vi "LC Language Demo.vi"() -> ()   [LabVIEW 2020]
uses:
  SubVI/LC Language.ctl
  SubVI/LC Single Control Information.ctl
  SubVI/LC Mode.ctl
  SubVI/LC Global Mode.ctl
panel:
  in  "Title":string="Language Change System"
  in  "Path":path
  in  "VI Path":string(tree)
  in  "Control Path":string(tree)
  in  "Import":bool
  in  "Export":bool
  in  "Class ID":u32
  in  "Control Type":string
  in  "Add":bool
  in  "Language":T1 items=["Chinese", "English"]
  in  "Property":u16(ring) items=["Blinking", "BoolText.Text", "Caption.Position", "Caption.Text", "Caption.Visible", "DefVal", "Desc", "FP.Title", "Lable.Text", "Lable.Visible", "Strings[4]", "TipStrip", "VI_Desc", "Visible"]
  in  "Control Ref":string
  in  "Control_Info":T2
  in  "Control List":i32(listbox)
  out "Time":string
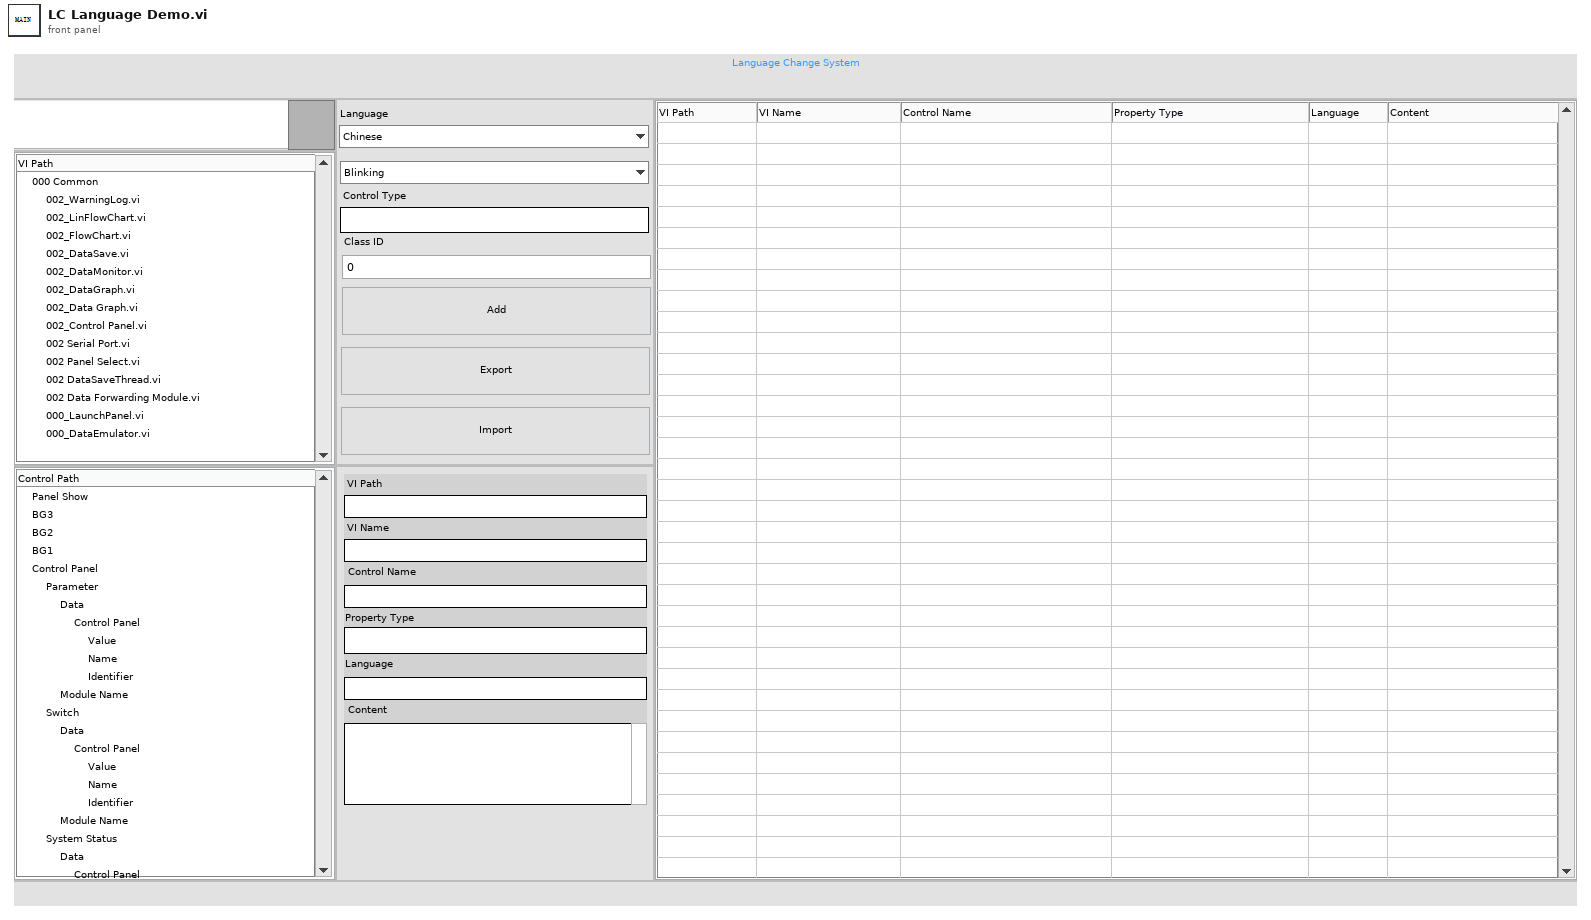
[diagram p1: front panel]
types:
  T1 = typedef "LC Language.ctl" = u16
  T2 = typedef "LC Single Control Information.ctl" = cluster{"VI Path":string, "VI Name":string, "Control Name":string, "Property Type":string, "Language":string, "Content":string}
  T3 = typedef "LC Global Mode.ctl" = enum16{"Init", "Read", "Write Language", "Write Version", "Save"}
  T4 = typedef "LC Mode.ctl" = enum16{"Init", "NONE", "Read", "Write", "Delete", "Clear", "Save"}
  T5 = typedef "LVPoint32TypeDef.ctl" = cluster{"Horizontal":i32, "Vertical":i32}
  T6 = typedef "LVRowAndColumnTypeDef.ctl" = cluster{"Row":i32, "Column":i32}
  T7 = enum32{"invalid app kind", "Development System", "Run Time System", "Student Edition", "Embedded LabVIEW", "Evaluation", "Custom"}
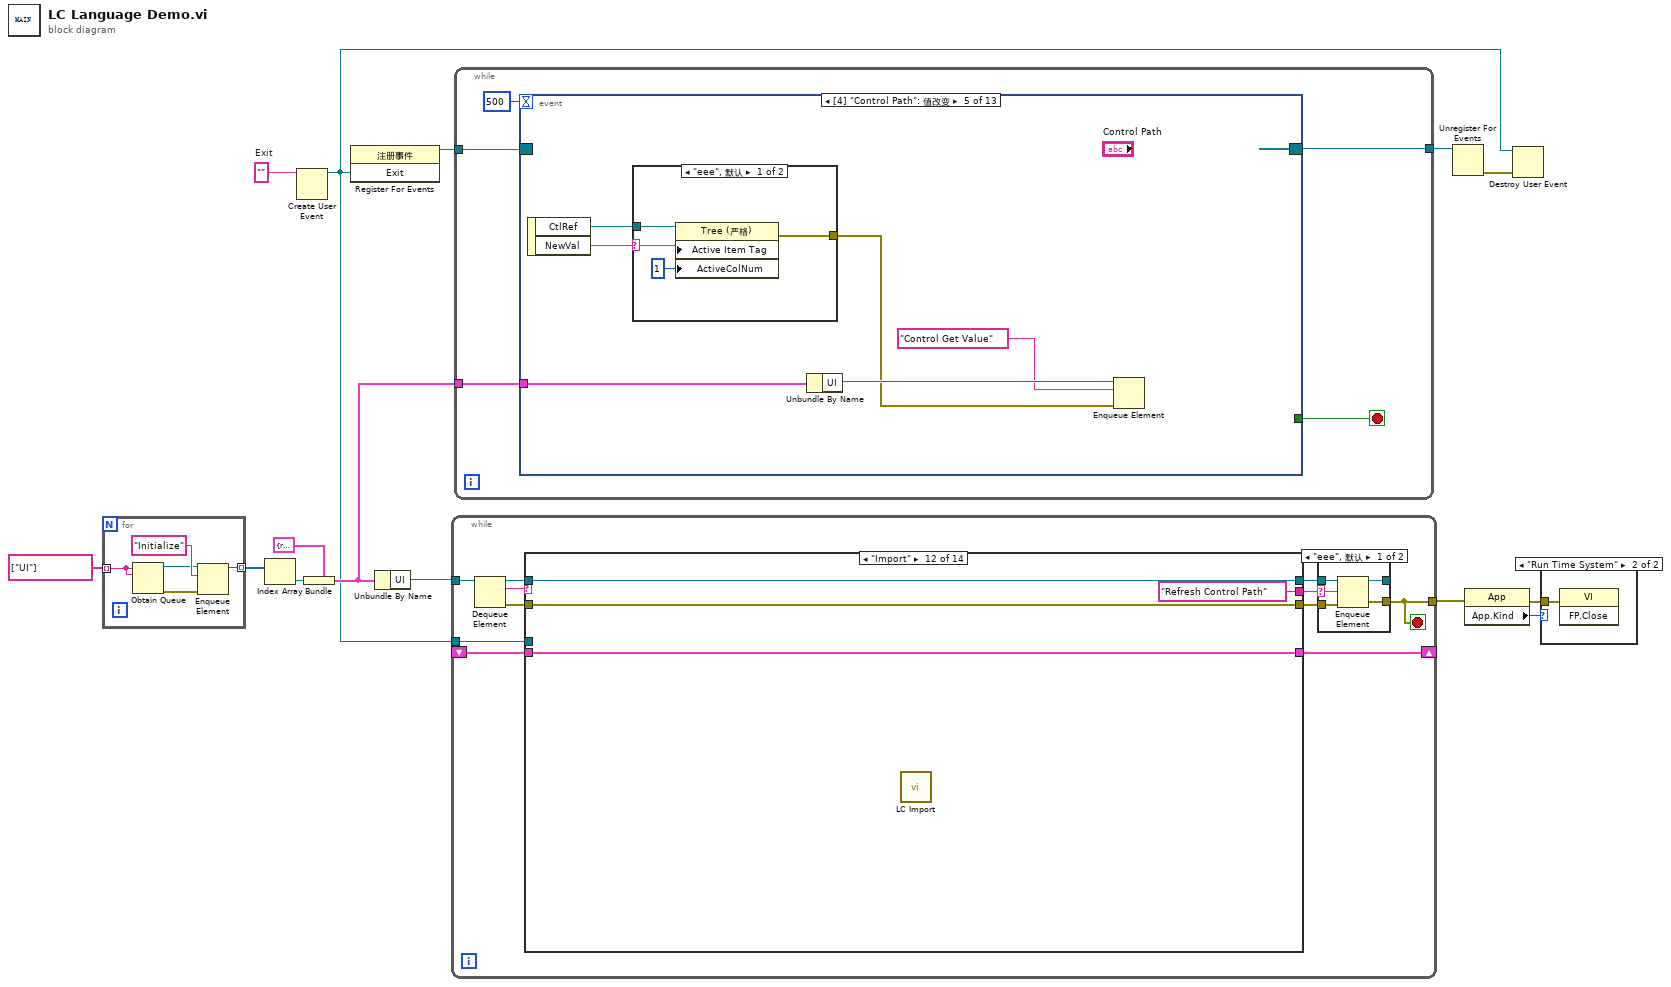
[diagram p0: block diagram]
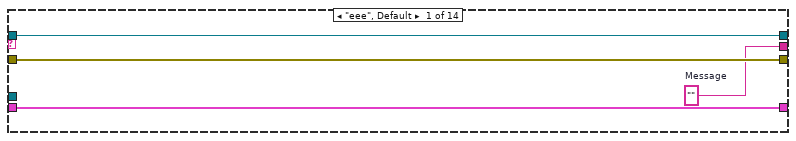
[diagram p4: hidden frame]
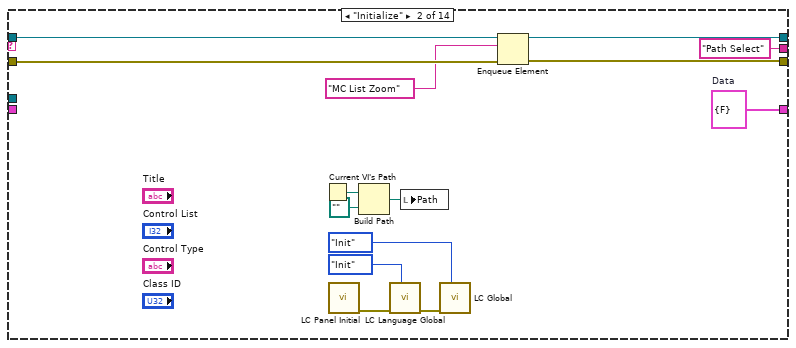
[diagram p5: hidden frame]
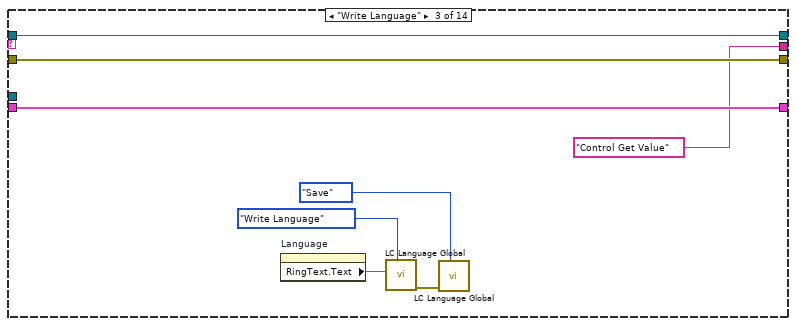
[diagram p6: hidden frame]
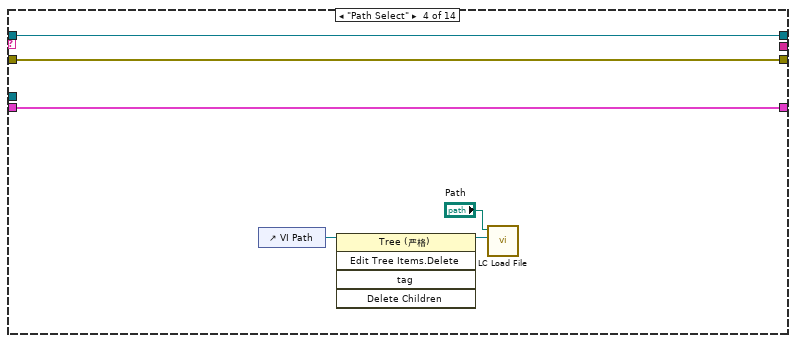
[diagram p7: hidden frame]
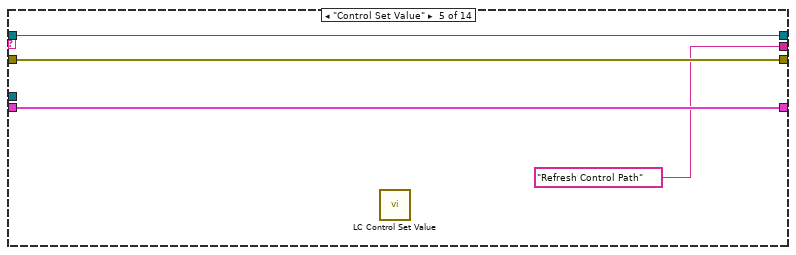
[diagram p8: hidden frame]
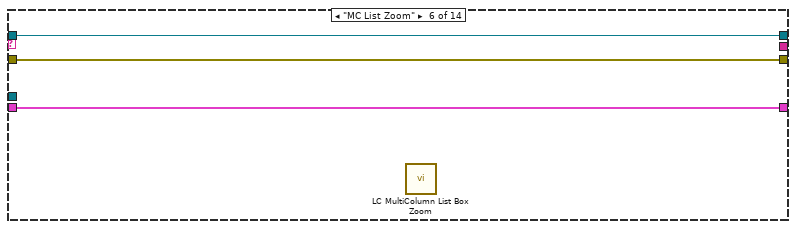
[diagram p9: hidden frame]
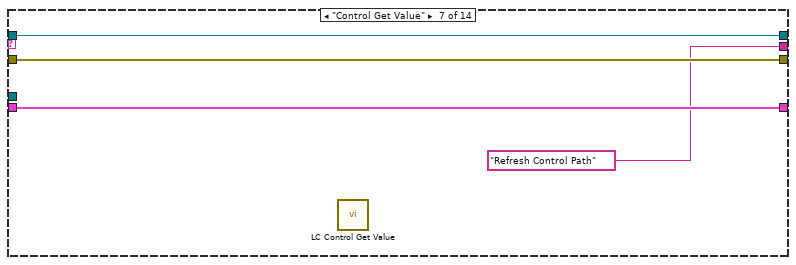
[diagram p10: hidden frame]
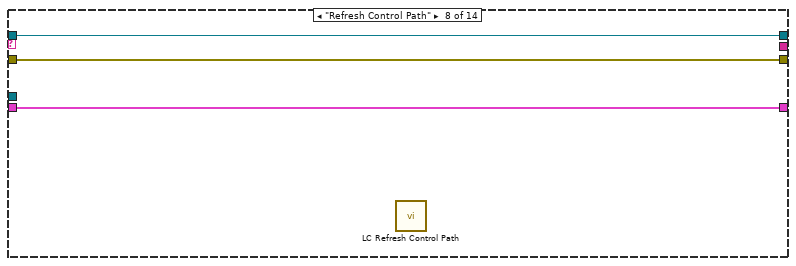
[diagram p11: hidden frame]
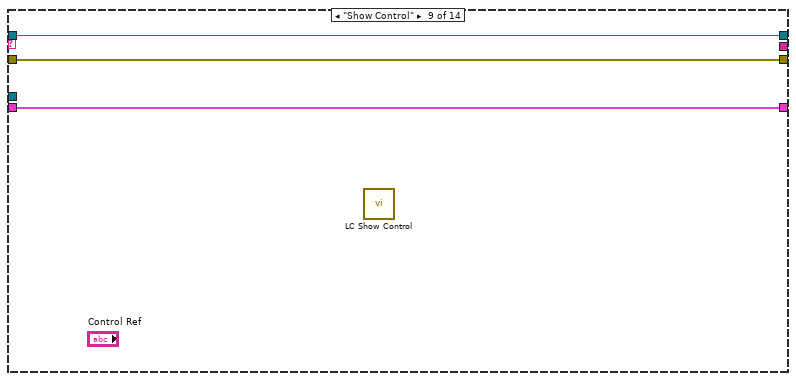
[diagram p12: hidden frame]
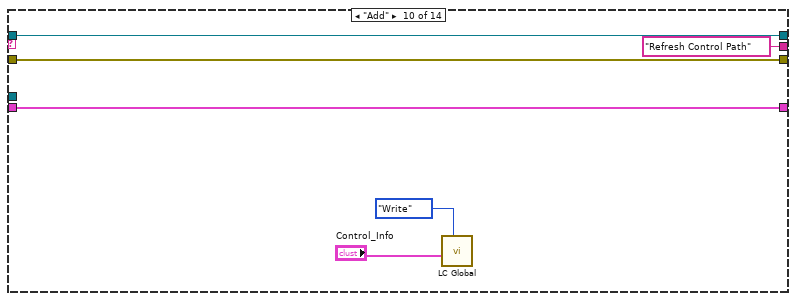
[diagram p13: hidden frame]
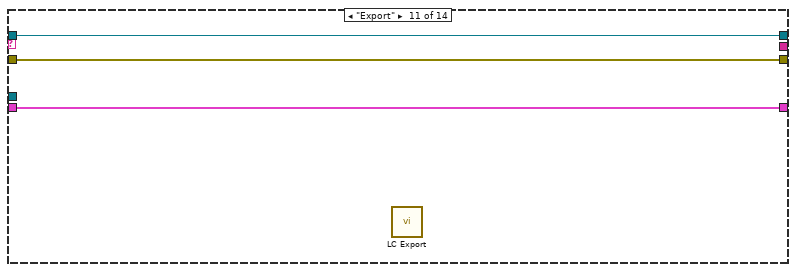
[diagram p14: hidden frame]
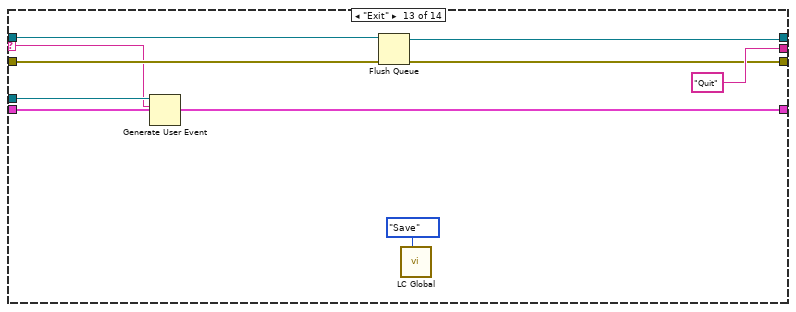
[diagram p15: hidden frame]
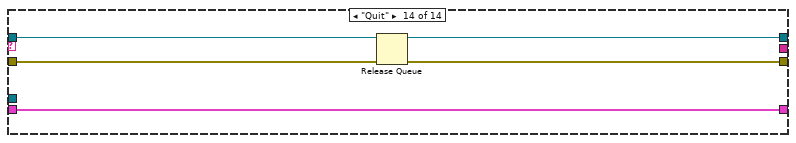
[diagram p16: hidden frame]
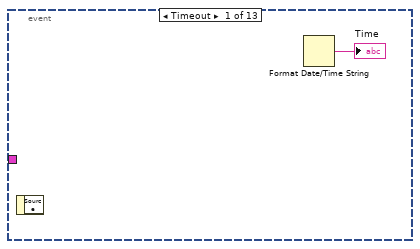
[diagram p17: hidden frame]
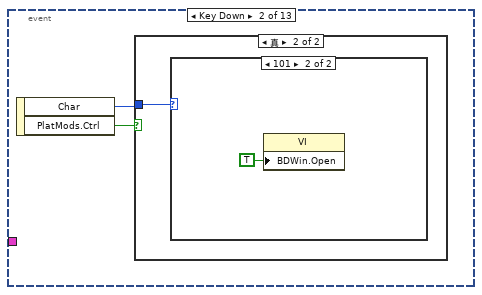
[diagram p18: hidden frame]
diagram:
  w4 = ""  # Exit
  n1 = for {
    tunnel: string[] ["UI"] -> [w15] mode=indexing
    tunnel: [w16] -> w9 mode=indexing
    n2 = Obtain Queue(name (unnamed)=w15, element data type=w15) -> (queue out=w18:refnum<queue>, error out=w17:errorcluster)  [unwired: 3 in, 1 out]
    n3 = Enqueue Element(queue=w18, element="Initialize" ("元素"), error in (no error)=w17) -> (queue out=w16:refnum<queue>)  [unwired: 1 in, 2 out]
  }
  n4 = Index Array(array=w9) -> (element=w13:refnum<queue>)  [unwired: 1 in]
  n5 = Create User Event(user event datatype=w4) -> (user event=w8:refnum<user-event>)  [unwired: 1 in, 1 out]
  n6 = Bundle(cluster=cluster{"UI":refnum<queue>} {"UI"=refnum}, "UI"=w13) -> (w14:cluster{"UI":refnum<queue>})
  n7 = register-events(w8) -> (reference out=w5:refnum<event-registration>)  [unwired: 2 in, 1 out]
  n8 = Unbundle By Name(w14) -> ("UI"=w10:refnum<queue>)
  n9 = while {
    tunnel: w10 -> [w30]
    tunnel: [w20] -> w1
    shift-right: [w24] -> _
    shift-left: _ -> [w23]
    tunnel: w8 -> [w22]
    stop <- w20 stop-if-true
    n10 = Dequeue Element(queue=w30) -> (queue out=w29:refnum<queue>, element=w21:string, error out=w26:errorcluster)  [unwired: 2 in, 1 out]
    n11 = case shown="\"Import\"" w21 {
      selector: w21 -> [_ _ _ _ _ _ _ _ _ _ _ _ w101 _]
      tunnel: w29 -> [w41 w47 w63 w69 w73 w76 w80 w83 w86 w92 w95 w99 w106 w112]
      tunnel: [w41 w44 w63 w69 w73 w76 w80 w83 w86 w92 w95 w99 w105 w112] -> w28
      tunnel: [w40 w43 w62 w68 w72 w75 w79 w82 w85 w91 w94 w98 w104 w109] -> w27
      tunnel: w26 -> [w40 w46 w62 w68 w72 w75 w79 w82 w85 w91 w94 w98 w103 w111]
      tunnel: [w39 "Path Select" ("Message") "Control Get Value" ("Message") _ "Refresh Control Path" ("Message") _ "Refresh Control Path" ("Message") _ _ "Refresh Control Path" ("Message") _ "Refresh Control Path" ("Message") "Quit" ("Message") _] -> w25
      tunnel: [w38 w55 w61 w67 w71 w74 w78 w81 w84 w90 w93 w97 w108 w110] -> w24
      tunnel: w23 -> [w38 _ w61 w67 w71 w74 w78 w81 w84 w90 w93 w97 w108 w110]
      tunnel: w22 -> [_ _ _ _ _ _ _ _ _ _ _ _ w102 _]
      frame "eee", Default {
        w39 = ""  # Message
      }
      frame "Initialize" {
        w55 = cluster{"Data":bool} {"Data"=FALSE}  # Data
        n12 = Current VI's Path() -> (path=w53:path)
        n13 = call "LC Panel Initial.vi"() -> ("error out"=w50:errorcluster)  [unwired: 11 in]
        n14 = Build Path(base path=w53, name or relative path=path ".." ("名称或相对路径")) -> (appended path=w51:path)
        n15 = call "LC Language Global.vi"("Mode"=LC_Global_Mode."Init", "error in (no error)"=w50) -> ("error out"=w49:errorcluster)  [unwired: 8 in, 1 out]
        n16 = local write "Path"(w51) -> ()
        n17 = call "LC Global.vi"("Mode"=LC_Mode."Init", "error in (no error)"=w49) -> ()  [unwired: 7 in, 3 out]
        n18 = Enqueue Element(queue=w47, element="MC List Zoom" ("元素"), error in (no error)=w46) -> (queue out=w44:refnum<queue>, error out=w43:errorcluster)  [unwired: 1 in, 1 out]
      }
      frame "Write Language" {
        n19 = property on="Language" class="Ring (严格)"() -> ("RingText.Text"=w59:string)  [unwired: 2 in, 2 out]
        n20 = call "LC Language Global.vi"("Mode"=LC_Global_Mode."Write Language", "String In"=w59) -> ("error out"=w57:errorcluster)  [unwired: 8 in, 1 out]
        n21 = call "LC Language Global.vi"("Mode"=LC_Global_Mode."Save", "error in (no error)"=w57) -> ()  [unwired: 8 in, 2 out]
      }
      frame "Path Select" {
        n22 = control-ref of="VI Path"() -> (w66:refnum<vi>)
        n23 = invoke class="Tree (严格)" method="Edit Tree Items.Delete"(reference=w66) -> (reference out=w65:refnum<vi>)  [unwired: 4 in, 4 out]
        n24 = call "LC Load File.vi"("VI Path"=w65, "selected path"="Path") -> ()  [unwired: 9 in, 1 out]
      }
      frame "Control Set Value" {
        n25 = call "LC Control Set Value.vi"() -> ()  [unwired: 11 in, 1 out]
      }
      frame "MC List Zoom" {
        n26 = call "LC MultiColumn List Box Zoom.vi"() -> ()  [unwired: 11 in, 1 out]
      }
      frame "Control Get Value" {
        n27 = call "LC Control Get Value.vi"() -> ()  [unwired: 11 in, 1 out]
      }
      frame "Refresh Control Path" {
        n28 = call "LC Refresh Control Path.vi"() -> ()  [unwired: 11 in, 1 out]
      }
      frame "Show Control" {
        n29 = call "LC Show Control.vi"() -> ()  [unwired: 11 in, 1 out]
      }
      frame "Add" {
        n30 = call "LC Global.vi"("Mode"=LC_Mode."Write", "Write"="Control_Info") -> ()  [unwired: 7 in, 3 out]
      }
      frame "Export" {
        n31 = call "LC Export.vi"() -> ()  [unwired: 11 in, 1 out]
      }
      frame "Import" {
        n32 = call "LC Import.vi"() -> ()  [unwired: 11 in, 1 out]
      }
      frame "Exit" {
        n33 = Generate User Event(user event=w102, event data cluster=w101) -> ()  [unwired: 2 in, 2 out]
        n34 = Flush Queue(queue=w106, error in (no error)=w103) -> (queue out=w105:refnum<queue>, error out=w104:errorcluster)  [unwired: 1 out]
        n35 = call "LC Global.vi"("Mode"=LC_Mode."Save") -> ()  [unwired: 8 in, 3 out]
      }
      frame "Quit" {
        n36 = Release Queue(queue=w112, error in (no error)=w111) -> (error out=w109:errorcluster)  [unwired: 1 in, 2 out]
      }
    }
    n37 = case shown="\"eee\", 默认" w25 {
      selector: w25 -> [w31 _]
      tunnel: w28 -> [w35 w37]
      tunnel: w27 -> [w34 w36]
      tunnel: [w33 w36] -> w20
      tunnel: [w32 w37] -> _
      frame "eee", Default {
        n38 = Enqueue Element(queue=w35, element=w31, error in (no error)=w34) -> (queue out=w32:refnum<queue>, error out=w33:errorcluster)  [unwired: 1 in, 1 out]
      }
      frame "" {
      }
    }
  }
  n39 = while {
    tunnel: w5 -> [w116]
    tunnel: [w115] -> w7
    tunnel: w14 -> [w114]
    stop <- w117 stop-if-true
    n40 = event shown="[4] \"Control Path\": 值改变" {
      selector: w116 -> [_ _ _ _ _ _ _ _ _ _ _ _ _]
      dyn-events: [_ _ _ _ _ _ _ _ _ _ _ _ _] -> w115
      timeout: 500 -> [_ _ _ _ _ _ _ _ _ _ _ _ _]
      tunnel: [_ _ w124 w129 _ _ _ _ _ _ _ _ _] -> w117
      tunnel: w114 -> [_ _ _ w128 w133 w144 w147 w150 w151 w163 w166 w169 _]
      event Timeout {
        n41 = event-data() -> ()  [unwired: 1 in, 1 out]
        n42 = Format Date/Time String() -> (date/time string=→"Time":string)  [unwired: 3 in]
      }
      event Key Down {
        n43 = event-data() -> ("Char"=w120:i16, "PlatMods.Ctrl"=w119:bool)  [unwired: 1 in]
        n44 = case shown="真" w119 {
          tunnel: w120 -> [_ w121]
          frame False {
          }
          frame True {
            n45 = case shown="101" w121 {
              frame 0, Default {
              }
              frame 101 {
                n46 = property class="VI"("BDWin.Open"=TRUE ("程序框图窗口:打开")) -> ()  [unwired: 2 in, 2 out]
              }
            }
          }
        }
      }
      event User Event {
        n47 = event-data() -> ("Exit"=w125:string)  [unwired: 1 in]
        n48 = Equal?(x=w125, y="Exit") -> (x = y?=w124:bool)
      }
      event Panel Close? {
        w129 = TRUE ("放弃？")
        n49 = event-data() -> ()  [unwired: 1 in, 1 out]
        n50 = Cluster To Array(cluster=w128) -> (array=w127:refnum<queue>[])
        n51 = for {
          tunnel: w127 -> [w131] mode=indexing
          tunnel: "Exit" ("元素") -> [w130]
          n52 = Enqueue Element(queue=w131, element=w130) -> ()  [unwired: 2 in, 3 out]
        }
        n53 = event-data("Discard?"=w129) -> ()  [unwired: 1 in, 1 out]
      }
      event "Control Path": Value Change {
        n54 = event-data() -> ("CtlRef"=w136:refnum<vi>, "NewVal"=w137:string)  [unwired: 1 in]
        n55 = case shown="\"eee\", 默认" w137 {
          selector: w137 -> [w139 _]
          tunnel: w136 -> [w140 _]
          tunnel: [w138 _] -> w132
          frame "eee", Default {
            n56 = property class="Tree (严格)"(reference=w140, "Active Item Tag"=w139, "ActiveColNum"=1 ("活动单元格:活动列数")) -> (error out=w138:errorcluster)  [unwired: 1 in, 1 out]
          }
          frame "" {
          }
        }
        n57 = Unbundle By Name(w133) -> ("UI"=w135:refnum<queue>)
        n58 = Enqueue Element(queue=w135, element="Control Get Value" ("元素"), error in (no error)=w132) -> ()  [unwired: 1 in, 3 out]
      }
      event "Path": Value Change {
        n59 = event-data() -> ()  [unwired: 1 in, 1 out]
        n60 = Unbundle By Name(w144) -> ("UI"=w143:refnum<queue>)
        n61 = Enqueue Element(queue=w143, element="Path Select" ("元素")) -> ()  [unwired: 2 in, 3 out]
      }
      event Value Change {
        n62 = event-data() -> ()  [unwired: 1 in, 6 out]
        n63 = Unbundle By Name(w147) -> ("UI"=w146:refnum<queue>)
        n64 = Enqueue Element(queue=w146, element="Control Set Value" ("元素")) -> ()  [unwired: 2 in, 3 out]
      }
      event Panel Resize {
        n65 = event-data() -> ()  [unwired: 1 in, 1 out]
        n66 = Unbundle By Name(w150) -> ("UI"=w149:refnum<queue>)
        n67 = Enqueue Element(queue=w149, element="MC List Zoom" ("元素")) -> ()  [unwired: 2 in, 3 out]
      }
      event "VI Path": Value Change {
        n68 = event-data() -> ("NewVal"=w156:string)  [unwired: 1 in]
        n69 = call <vilib>:"Delimited String to 1D String Array.vi"("delimiter"=".", "delimited string"=w156) -> ("string array"=w154:string[])  [unwired: 9 in]
        n70 = Index Array(array=w154, index=1 ("索引")) -> (element=w152:string)
        n71 = case shown="\"vi\"" w152 {
          tunnel: w151 -> [_ w159]
          frame "eee", Default {
          }
          frame "vi" {
            n72 = Unbundle By Name(w159) -> ("UI"=w158:refnum<queue>)
            n73 = Enqueue Element(queue=w158, element="Refresh Control Path" ("元素")) -> ()  [unwired: 2 in, 3 out]
          }
        }
      }
      event "Add", "Export", "Import": Value Change {
        n74 = event-data() -> ("CtlRef"=w161:refnum<vi>)  [unwired: 1 in]
        n75 = Unbundle By Name(w163) -> ("UI"=w162:refnum<queue>)
        n76 = property class="Bool"(reference=w161) -> ("Label.Text"=w160:string)  [unwired: 1 in, 2 out]
        n77 = Enqueue Element(queue=w162, element=w160) -> ()  [unwired: 2 in, 3 out]
      }
      event Value Change {
        n78 = event-data() -> ()  [unwired: 1 in, 1 out]
        n79 = Unbundle By Name(w166) -> ("UI"=w165:refnum<queue>)
        n80 = Enqueue Element(queue=w165, element="Write Language" ("元素")) -> ()  [unwired: 2 in, 3 out]
      }
      event "Property": Value Change {
        n81 = event-data() -> ()  [unwired: 1 in, 1 out]
        n82 = Unbundle By Name(w169) -> ("UI"=w168:refnum<queue>)
        n83 = Enqueue Element(queue=w168, element="Control Get Value" ("元素")) -> ()  [unwired: 2 in, 3 out]
      }
      event "Control List": Mouse Down {
        n84 = event-data() -> ("CtlRef"=w174:refnum<vi>, "Coords"=w173:T5)  [unwired: 1 in]
        n85 = invoke class="MCListbox (严格)" method="Point To Row Column"(reference=w174, "Point"=w173) -> (reference out=w170:refnum<vi>, "CellPosition"=w172:T6)  [unwired: 5 in, 5 out]
        n86 = Unbundle(w172) -> ("Row"=w171:i32)  [unwired: 1 out]
        n87 = property class="MCListbox (严格)"(reference=w170, "Value"=w171) -> ()  [unwired: 1 in, 2 out]
      }
    }
  }
  n88 = Unregister For Events(event registration refnum=w7) -> (error out=w6:errorcluster)  [unwired: 1 in]
  n89 = property class="App"(error in=w1) -> (error out=w2:errorcluster, "App.Kind"=w3:T7)  [unwired: 1 in, 1 out]
  n90 = Destroy User Event(user event=w8, error in=w6) -> ()  [unwired: 1 out]
  n91 = case shown="\"Run Time System\"" w3 {
    tunnel: w2 -> [_ w175]
    frame "invalid app kind", Default {
    }
    frame "Run Time System" {
      n92 = invoke class="VI" method="FP.Close"(error in=w175) -> ()  [unwired: 2 in, 3 out]
    }
  }
